vi "Limelight Snapshot ON & OFF.vi"(11 "ON & OFF":bool) -> (0 "error out":errorcluster)   [LabVIEW 2019]
uses:
  <vilib>/Rock Robotics/Network Tables/NT Write Number.vi
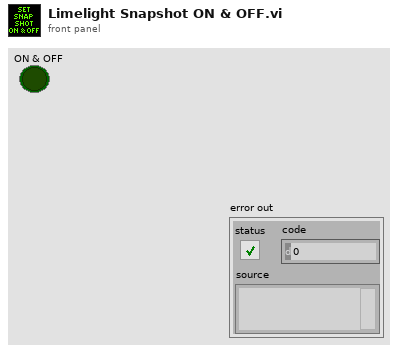
[diagram p1: front panel]
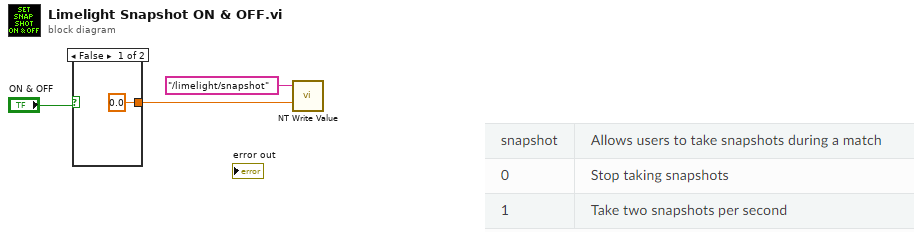
[diagram p0: block diagram]
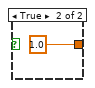
[diagram p2: hidden frame]
diagram:
  n1 = case shown="False" "ON & OFF" {
    tunnel: [0.0 ("Numeric") 1.0 ("Numeric")] -> w2
    frame False {
    }
    frame True {
    }
  }
  n2 = call-poly <vilib>:"NT Write Value.vi"("Numeric"=w2, "Name"="/limelight/snapshot") -> ()  [unwired: 9 in, 1 out]
